vi "Query Range Test.vi"(8 "error in (no error)":errorcluster, 10 "Calculate Block (1: Calculate Block 1)":i32(ring)=1 items=["Calculate Block 1"=1, "Calculate Block 2"=2, "Calculate Block 3"=3, "Calculate Block 4"=4], 11 "VISA resource name":refnum<visa-resource-name>) -> (0 "error out":errorcluster, 1 "Limit Failure?":bool, 2 "Failure Count":i32, 3 "VISA resource name out":refnum<visa-resource-name>)   [LabVIEW 2018, in "Agilent U2000 Series.lvlib"]
doc: "Queries the instrument to determine if the upper or lower limit has been exceeded. The properties of the range can be configured by calling the Configure Range VI."
uses:
  Agilent U2000 Series.lvlib
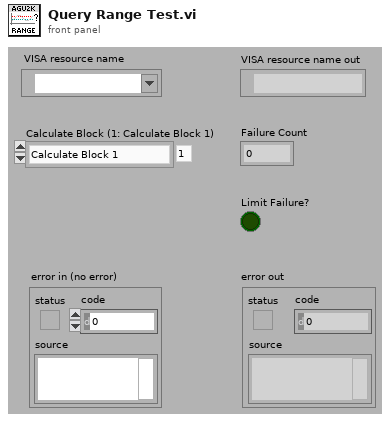
[diagram p1: front panel]
types:
  T1 = typedef "Agilent U2000 Series.lvlib/Extended User Data.ctl" = cluster{"U2000 Series Mode":u16, "Trigger Source Int/Ext":bool}
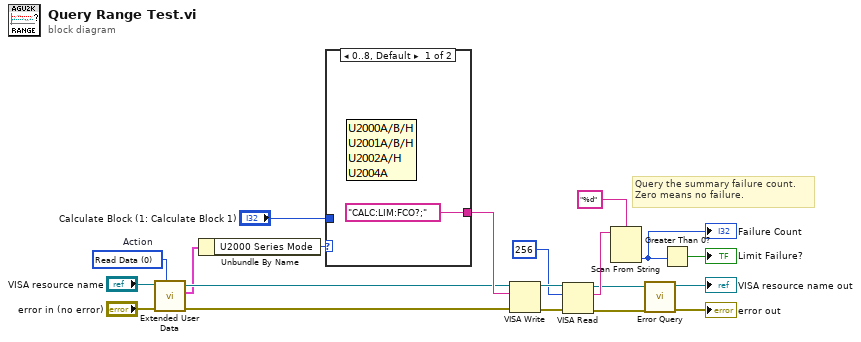
[diagram p0: block diagram]
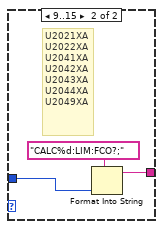
[diagram p2: hidden frame]
diagram:
  w3 = 0 items=["Read Data", "Write Data", "Clear Data", "Clear ALL Data"]  # Action
  # "Query the summary failure count.\nZero means no failure."
  n1 = call "Extended User Data.vi"("Action (1: Write Data)"=w3, "error in (no error)"="error in (no error)", "VISA resource name"="VISA resource name") -> ("error out"=w5:errorcluster, "User Data Out"=w2:T1, "VISA resource name out"=w4:refnum<visa-resource-name>)  [unwired: 1 in, 5 out]
  n2 = Unbundle By Name(w2) -> ("U2000 Series Mode"=w1:u16)
  n3 = case shown="0..8, Default" w1 {
    tunnel: "Calculate Block (1: Calculate Block 1)" -> [_ w24]
    tunnel: ["CALC:LIM:FCO?;" w22] -> w8
    frame 0..8, Default {
    }
    frame 9..15 {
      # "U2021XA\nU2022XA\nU2041XA\nU2042XA\nU2043XA\nU2044XA\nU2049XA"
      n4 = Format Into String(format string="CALC%d:LIM:FCO?;", w24) -> (resulting string=w22:string)  [unwired: 2 in, 1 out]
    }
  }
  n5 = VISA Write(VISA resource name=w4, write buffer=w8, error in (no error)=w5) -> (VISA resource name out=w19:refnum<visa-resource-name>, error out=w20:errorcluster)  [unwired: 1 out]
  n6 = VISA Read(VISA resource name=w19, byte count=u32 256, error in (no error)=w20) -> (VISA resource name out=w12:refnum<visa-resource-name>, read buffer=w17:string, error out=w11:errorcluster)  [unwired: 1 out]
  n7 = Scan From String(format string="%d", input string=w17) -> (output 1=w14:i32)  [unwired: 2 in, 4 out]
  "Failure Count" <- w14
  n8 = call "Error Query.vi"("error in (no error)"=w11, "VISA resource name"=w12) -> ("error out"=→"error out":errorcluster, "VISA resource name out"=→"VISA resource name out":refnum<visa-resource-name>)  [unwired: 8 out]
  n9 = Greater Than 0?(x=w14) -> (x > 0?=→"Limit Failure?":bool)
